vi "Validate Routing Channel Parameters.vi"(6 "initial state":string="No Connections", 8 "error in":errorcluster, 9 "state configurations":T1=[{"Name"="No Connections", "Description"="State with no connections", "Value"=-1, "Connection List"=[]}], 10 "channel name":string, 11 "routing channels in":T4 format="%.0x") -> (0 "error out":errorcluster, 3 "routing channels out":T4 format="%.0x")   [LabVIEW 2017, in "Routing and Faulting Scripting.lvlib"]
uses:
  Routing and Faulting Scripting.lvlib
  <vilib>/NI Veristand/Custom Device API/Custom Device Item Ref.ctl
  Shared/Channel States.ctl
  Shared/Routing State.ctl
  Shared/Connection.ctl
  <vilib>/NI Veristand/Custom Device API/Custom Device API.lvlib
  Shared/Routing and Faulting Shared.lvlib
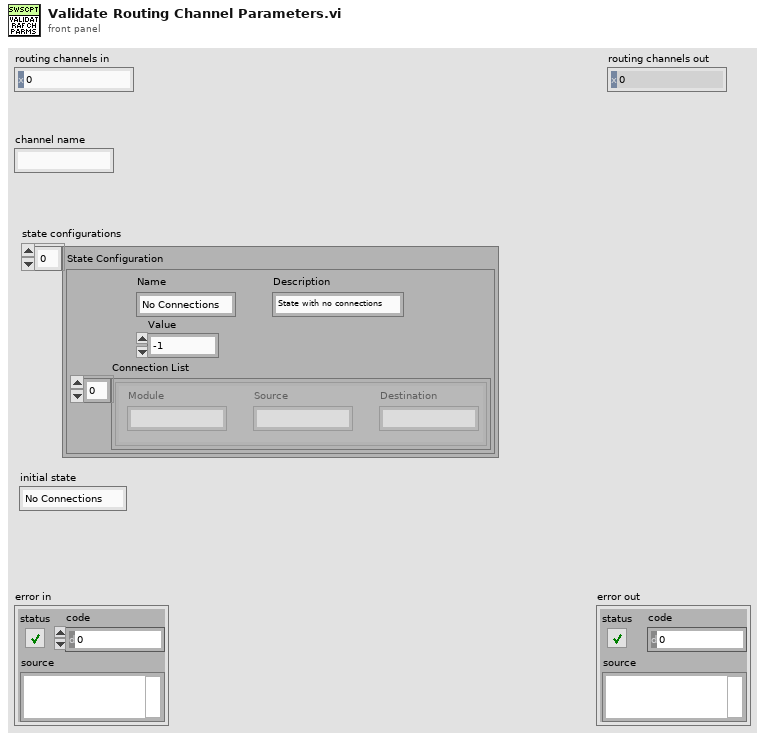
[diagram p1: front panel]
types:
  T1 = typedef "Routing and Faulting Shared.lvlib/Channel States.ctl" = T2[]
  T2 = typedef "Routing and Faulting Shared.lvlib/Routing State.ctl" = cluster{"Name":string, "Description":string, "Value":i32, "Connection List":T3[]}
  T3 = typedef "Routing and Faulting Shared.lvlib/Connection.ctl" = cluster{"Module":string, "Source":string, "Destination":string}
  T4 = typedef "Custom Device API.lvlib/Custom Device Item Ref.ctl" = u64
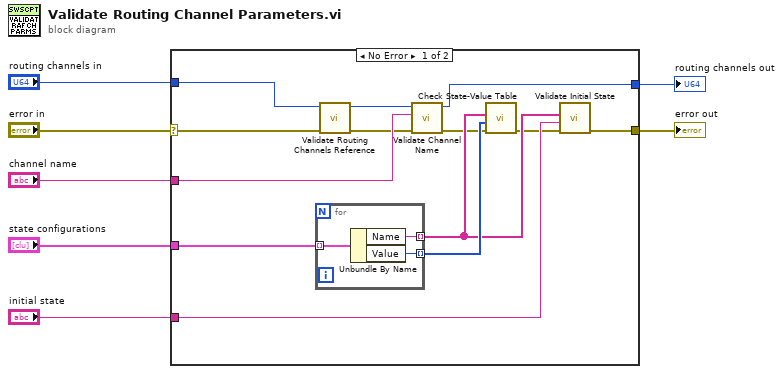
[diagram p0: block diagram]
diagram:
  n1 = case shown="No Error" "error in" {
    selector: "error in" -> [w11 w25]
    tunnel: [w12 w25] -> w7
    tunnel: "routing channels in" -> [w9 w24]
    tunnel: "channel name" -> [w18 _]
    tunnel: "state configurations" -> [w20 _]
    tunnel: "initial state" -> [w16 _]
    tunnel: [w17 w24] -> w1
    frame No Error {
      n2 = for {
        tunnel: w20 -> [w23] mode=indexing
        tunnel: [w22] -> w15 mode=indexing
        tunnel: [w21] -> w19 mode=indexing
        n3 = Unbundle By Name(w23) -> ("Name"=w22:string, "Value"=w21:i32)
      }
      n4 = call "Validate Routing Channels Reference.vi"("error in (no error)"=w11, "Routing Channels Ref in"=w9) -> ("error out"=w10:errorcluster, "Routing Channels Ref out"=w8:T4)  [unwired: 8 in]
      n5 = call "Validate Channel Name.vi"("error in (no error)"=w10, "Channel Name"=w18, "Routing Channels Ref in"=w8) -> ("error out"=w13:errorcluster, "Parent Ref out"=w17:T4)  [unwired: 7 in]
      n6 = call "Check State-Value Table.vi"("error in (no error)"=w13, "State Values"=w19, "State Names"=w15) -> ("error out"=w14:errorcluster)  [unwired: 7 in, 1 out]
      n7 = call "Validate Initial State.vi"("error in (no error)"=w14, "Intial State"=w16, "State Names"=w15) -> ("error out"=w12:errorcluster)  [unwired: 7 in, 1 out]
    }
    frame Error {
    }
  }
  "error out" <- w7
  "routing channels out" <- w1
